vi "UpdateLifetime.vi"(10 "Lifecycle":T1, 11 "Actor":refnum<class "Actor.lvclass">) -> (3 "Actor":refnum<class "Actor.lvclass">)   [LabVIEW 2020, in "jettl.lvlib"]
uses:
  jettl.lvlib
  Actor/Actor.lvclass
  Lifecycle.ctl
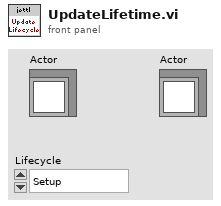
[diagram p1: front panel]
types:
  T1 = typedef "jettl.lvlib/Lifecycle.ctl" = enum16{"Setup", "TeardownBeforeStart", "Start", "Running", "Stop", "TeardownAfterStart"}
  T2 = typedef "jettl.lvlib/Base.ctl" = cluster{"Lifecycle":T1, "SelfActor":T3, "MediatorActor":T3, "ComponentActorMap":T8}
  T3 = typedef "jettl.lvlib/Actor.ctl" = cluster{"Messages":T4, "ActorAlias":string, "ActorType":T7, "Transport":refnum<user-event>, "EventRegistrationRef":refnum<event-registration>, "VIRef":refnum<vi>}
  T4 = typedef "jettl.lvlib/Messages.ctl" = cluster{"Listen":T5, "TellSelf":T5, "TellMediator":T5, "TellComponentMap":T6}
  T5 = typedef "jettl.lvlib/MessageSet.ctl" = set{refnum<class "Message.lvclass">}
  T6 = typedef "jettl.lvlib/TellComponentMap.ctl" = map{string, T5}
  T7 = typedef "jettl.lvlib/ActorType.ctl" = enum16{"Mediator", "Component"}
  T8 = typedef "jettl.lvlib/ComponentActorMap.ctl" = map{string, T3}
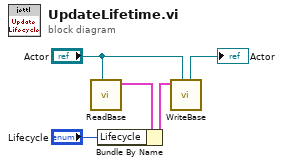
[diagram p0: block diagram]
diagram:
  n1 = call-dynamic "ReadBase.vi"("Actor"="Actor") -> ("Base"=w5:T2)  [unwired: 10 in]
  n2 = Bundle By Name(cluster=w5, "Lifecycle"="Lifecycle") -> (w4:T2)
  n3 = call-dynamic "WriteBase.vi"("Actor"="Actor", "Base"=w4) -> ("Actor"=→"Actor":refnum<class "Actor.lvclass">)  [unwired: 9 in]
